vi "Teleop.vi"(10 "Match Info":T1={"Autonomous Elapsed Seconds"=0.0, "TeleOp Elapsed Seconds"=0.0, "Disabled Elapsed Seconds"=0.0, "Visited Autonomous"=FALSE, "Visited TeleOp"=FALSE, "Visited Disabled"=FALSE, "Autonomous Settings"={"Autonomous Style"=enum."Independent", "VI Refnum"=refnum}}, 11 "Call Context":T2) -> ()   [LabVIEW 2016]
doc: "This VI is called for each TeleOp packet received from the DS where the robot is not disabled. It is often used to read from the joysticks and update I/O or to update setpoints for timed control loops. It should complete and return within 20 milliseconds or it may miss DS packets."
uses:
  <vilib>/Rock Robotics/WPI/DriverStation/WPI_DriverStationDerivedRobotMode.ctl
  <vilib>/Rock Robotics/WPI/DriverStation/WPI_DriverStationMatch Info.ctl
  <vilib>/Rock Robotics/WPI/Utilities/WPI_GetSetVariantRefNum.vi
  <vilib>/Rock Robotics/Network Tables/NT Write Boolean Array.vi
  <vilib>/Rock Robotics/Network Tables/NT Write Numeric Array.vi
  <vilib>/Rock Robotics/Network Tables/NT Read Boolean.vi
  <vilib>/Rock Robotics/Network Tables/NT Read Number.vi
panel:
  out "Sample Slider 0":dbl(slide) scale=0.0..5.0
  out "Sample Boolean 1":bool
  out "Sample Boolean 0":bool
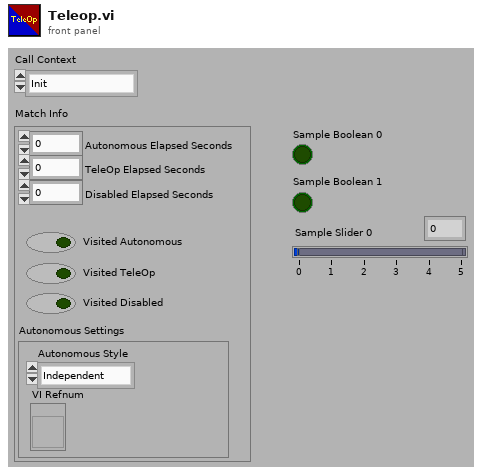
[diagram p1: front panel]
types:
  T1 = typedef "WPI_DriverStationMatch Info.ctl" = cluster{"Autonomous Elapsed Seconds":dbl, "TeleOp Elapsed Seconds":dbl, "Disabled Elapsed Seconds":dbl, "Visited Autonomous":bool, "Visited TeleOp":bool, "Visited Disabled":bool, "Autonomous Settings":cluster{"Autonomous Style":enum16{"Iterative", "Independent"}, "VI Refnum":refnum<vi>}}
  T2 = typedef "WPI_DriverStationDerivedRobotMode.ctl" = enum16{"Init", "Execute", "Stop"}
  T3 = typedef "WPI_JoystickDevRef.ctl" = cluster{"Device":T4}
  T4 = typedef "WPI_JoystickDeviceEnum.ctl" = enum16{"USB 0", "USB 1", "USB 2", "USB 3", "USB 4", "USB 5"}
  T5 = typedef "WPI_RobotDriveDevRef.ctl" = cluster{"DevStatus":errorcluster, "Motors[]":T6[], "Square Inputs":bool, "Max Output":dbl}
  T6 = typedef "WPI_MotorControlDeviceRef.ctl" = cluster{"DeviceStatus":errorcluster, "Type":T7, "PWM":cluster{"PWM Channel":T8, "DeadBand":T9}, "CAN":cluster{"Device Number":u8, "SetOutput VI Ref":variant, "GetOutput VI Ref":variant, "Enable VI Ref":variant, "Disable VI Ref":variant, "Data":variant}, "Invert":bool}
  T7 = typedef "WPI_MotorControlType.ctl" = enum16{"PWM", "CAN"}
  T8 = typedef "FPGA_DIOPWMChannel.ctl" = enum8{"PWM 0", "PWM 1", "PWM 2", "PWM 3", "PWM 4", "PWM 5", "PWM 6", "PWM 7", "PWM 8", "PWM 9", "PWM MXP 0", "PWM MXP 1", "PWM MXP 2", "PWM MXP 3", "PWM MXP 4", "PWM MXP 5", "PWM MXP 6", "PWM MXP 7", "PWM MXP 8", "PWM MXP 9", "Invalid"}
  T9 = typedef "WPI_PWMDeadband.ctl" = cluster{"Name":string, "maxPositivePwm":i32, "minPositivePwm":i32, "centerPwm":i32, "maxNegativePwm":i32, "minNegativePwm":i32, "angularRange":u16}
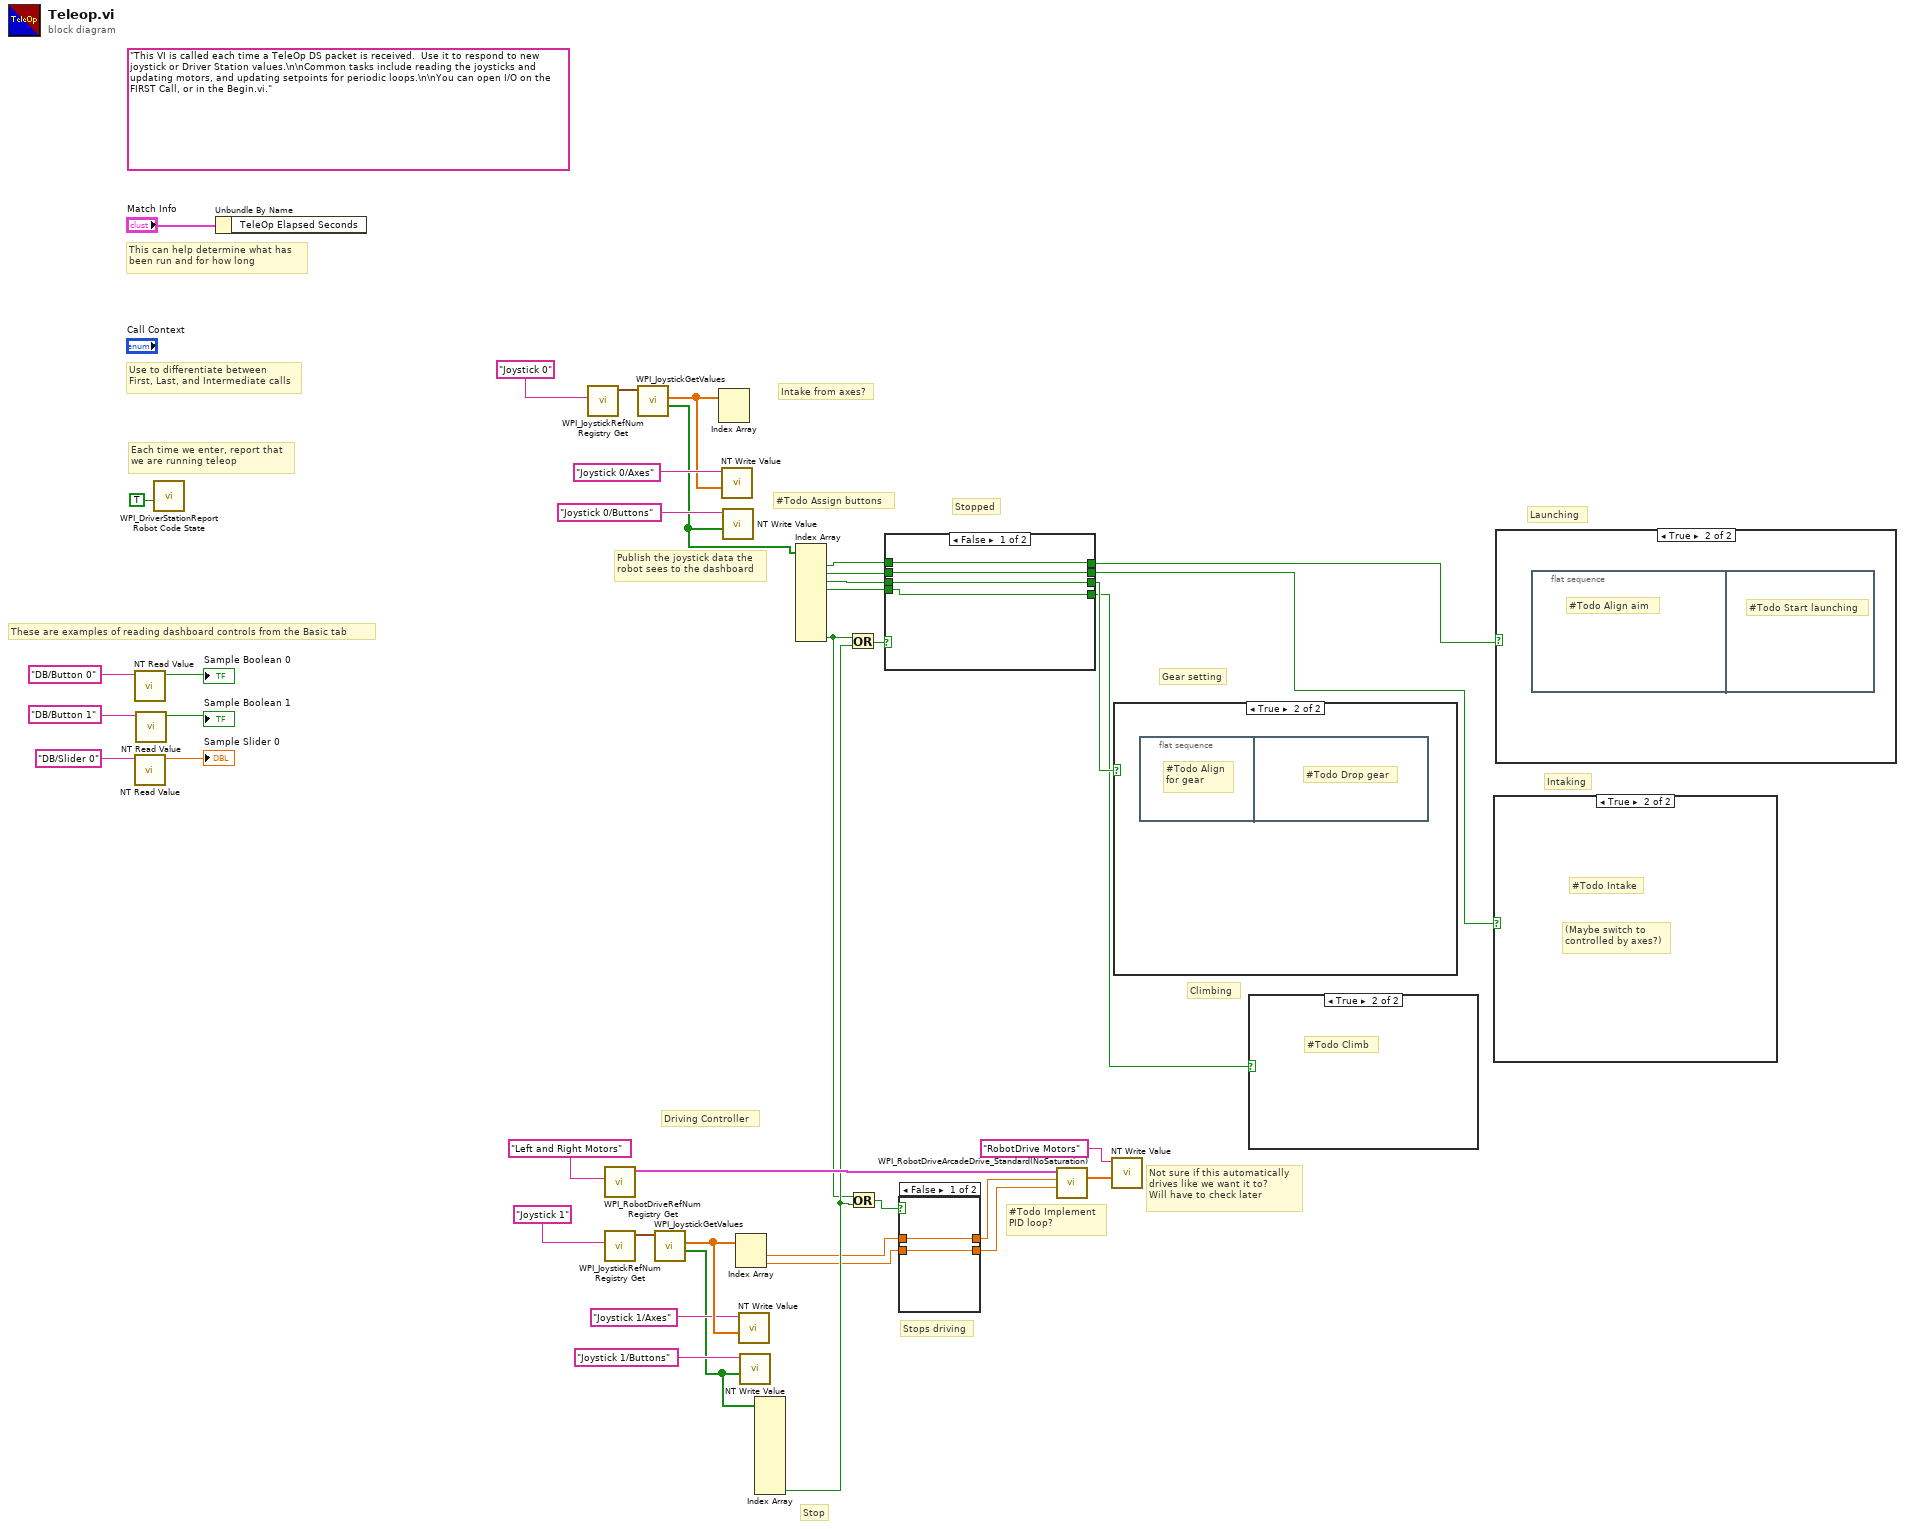
[diagram p0: block diagram]
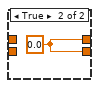
[diagram p3: hidden frame]
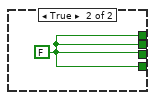
[diagram p4: hidden frame]
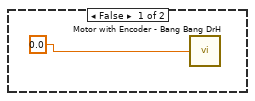
[diagram p7: hidden frame]
diagram:
  (unwired) "This VI is called each time a TeleOp DS packet is received.  Use it to respond to new joystick or Driver Station values.\n\nCommon tasks include reading the joysticks and updating motors, and updating setpoints for periodic loops.\n\nYou can open I/O on the FIRST Call, or in the Begin.vi."
  # "Climbing"
  # "#Todo Implement\nPID loop?"
  # "Stops driving"
  # "Not sure if this automatically\ndrives like we want it to?\nWill have to check later"
  # "Stop"
  # "Stopped"
  # "Gear setting"
  # "Intake from axes?"
  # "Driving Controller"
  # "#Todo Assign buttons"
  # "Intaking"
  # "Launching"
  # "These are examples of reading dashboard controls from the Basic tab"
  # "Publish the joystick data the\nrobot sees to the dashboard"
  # "Each time we enter, report that\nwe are running teleop"
  # "Use to differentiate between\nFirst, Last, and Intermediate calls"
  # "This can help determine what has\nbeen run and for how long"
  n1 = call-poly <vilib>:"NT Read Value.vi"("Name"="DB/Button 0" ("refnum name")) -> ("Boolean"=→"Sample Boolean 0":bool)  [unwired: 9 in, 1 out]
  n2 = call-poly <vilib>:"NT Read Value.vi"("Name"="DB/Slider 0" ("refnum name")) -> ("Numeric"=→"Sample Slider 0":dbl)  [unwired: 9 in, 1 out]
  n3 = call-poly <vilib>:"NT Read Value.vi"("Name"="DB/Button 1" ("refnum name")) -> ("Boolean"=→"Sample Boolean 1":bool)  [unwired: 9 in, 1 out]
  n4 = call <vilib>:"WPI_DriverStationReport Robot Code State.vi"("TeleOp"=TRUE ("Autonomous")) -> ()  [unwired: 10 in, 1 out]
  n5 = Unbundle By Name("Match Info") -> ()  [unwired: 1 out]
  n6 = call <vilib>:"WPI_JoystickRefNum Registry Get.vi"("refnum name"="Joystick 0") -> ("JoystickDevRef"=w38:T3)  [unwired: 1 in, 9 out]
  n7 = call <vilib>:"WPI_RobotDriveRefNum Registry Get.vi"("refnum name"="Left and Right Motors") -> ("RobotDriveDevRef"=w20:T5)  [unwired: 1 in, 9 out]
  n8 = call <vilib>:"WPI_JoystickRefNum Registry Get.vi"("refnum name"="Joystick 1") -> ("JoystickDevRef"=w22:T3)  [unwired: 1 in, 9 out]
  n9 = call <vilib>:"WPI_JoystickGetValues.vi"("JoystickDevRef"=w38) -> ("Buttons"=w18:bool[], "Axes"=w34:dbl[])  [unwired: 6 in, 3 out]
  n10 = call <vilib>:"WPI_JoystickGetValues.vi"("JoystickDevRef"=w22) -> ("Buttons"=w11:bool[], "Axes"=w25:dbl[])  [unwired: 6 in, 3 out]
  n11 = Index Array(array=w34) -> ()  [unwired: 2 in, 2 out]
  n12 = call-poly <vilib>:"NT Write Value.vi"("Numeric Array"=w34, "Name"="Joystick 0/Axes") -> ()  [unwired: 9 in, 1 out]
  n13 = call-poly <vilib>:"NT Write Value.vi"("Boolean Array"=w18, "Name"="Joystick 0/Buttons") -> ()  [unwired: 9 in, 1 out]
  n14 = Index Array(array=w25) -> (element #1=w6:dbl, element #2=w5:dbl)  [unwired: 2 in]
  n15 = call-poly <vilib>:"NT Write Value.vi"("Numeric Array"=w25, "Name"="Joystick 1/Axes") -> ()  [unwired: 9 in, 1 out]
  n16 = call-poly <vilib>:"NT Write Value.vi"("Boolean Array"=w11, "Name"="Joystick 1/Buttons") -> ()  [unwired: 9 in, 1 out]
  n17 = Index Array(array=w11) -> (element #10=w8:bool)  [unwired: 10 in, 9 out]
  n18 = Index Array(array=w18) -> (element #1=w16:bool, element #2=w14:bool, element #3=w12:bool, element #4=w2:bool, element #10=w7:bool)  [unwired: 10 in, 5 out]
  n19 = Or(x=w7, y=w8) -> (x .or. y?=w10:bool)
  n20 = Or(x=w7, y=w8) -> (x .or. y?=w9:bool)
  n21 = case shown="False" w10 {
    tunnel: [w44 w45] -> w17
    tunnel: w16 -> [w44 _]
    tunnel: [w43 w45] -> w15
    tunnel: w14 -> [w43 _]
    tunnel: [w42 w45] -> w13
    tunnel: w12 -> [w42 _]
    tunnel: w2 -> [w41 _]
    tunnel: [w41 w45] -> w1
    frame False {
    }
    frame True {
      w45 = FALSE
    }
  }
  n22 = case shown="False" w9 {
    tunnel: w6 -> [w47 _]
    tunnel: w5 -> [w46 _]
    tunnel: [w47 w48] -> w4
    tunnel: [w46 w48] -> w3
    frame False {
    }
    frame True {
      w48 = 0.0
    }
  }
  n23 = call <vilib>:"WPI_RobotDriveArcadeDrive_Standard(NoSaturation).vi"("Y axis value"=w3, "X axis value"=w4, "RobotDriveDevRef"=w20) -> ("Motor Values"=w26:dbl[])  [unwired: 1 in, 7 out]
  n24 = call-poly <vilib>:"NT Write Value.vi"("Numeric Array"=w26, "Name"="RobotDrive Motors") -> ()  [unwired: 9 in, 1 out]
  n25 = case shown="True" w13 {
    frame False {
    }
    frame True {
      n26 = flat-sequence {
        frame #0 {
          # "#Todo Align\nfor gear"
        }
        frame #1 {
          # "#Todo Drop gear"
        }
      }
    }
  }
  n27 = case shown="True" w1 {
    frame False {
    }
    frame True {
      # "#Todo Climb"
    }
  }
  n28 = case shown="True" w15 {
    frame False {
    }
    frame True {
      # "(Maybe switch to \ncontrolled by axes?)"
      # "#Todo Intake"
    }
  }
  n29 = case shown="True" w17 {
    frame False {
      n30 = call "Motor with Encoder - Bang Bang DrH.vi"("Target RPM"=0.0) -> ()  [unwired: 1 in]
    }
    frame True {
      n31 = flat-sequence {
        frame #0 {
          # "#Todo Align aim"
        }
        frame #1 {
          # "#Todo Start launching"
        }
      }
    }
  }
